vi "_io_get_StatusByte.vi"(5 "Block Setting of VISA Timeout for viReadSTB":bool, 7 "Method (viReadSTB)":u16(ring) items=["viReadSTB", "*STB?"], 8 "error in":errorcluster caption="error in (no error)", 10 "Bits filter (None - 0xFF)":u16=255 format="%.0x", 11 "VISA resource name":refnum<visa-resource-name>) -> (0 "error out":errorcluster, 1 "Error":bool, 2 "STB returned":u16 format="%.0x", 3 "VISA resource name out":refnum<visa-resource-name>, 4 "MAV":bool, 6 "OPC (ESB)":bool)   [LabVIEW 2020, in "Rohde&Schwarz RTx Oscilloscopes.lvlib" / "rsidr_core.lvlib"]
uses:
  rsidr_core.lvlib
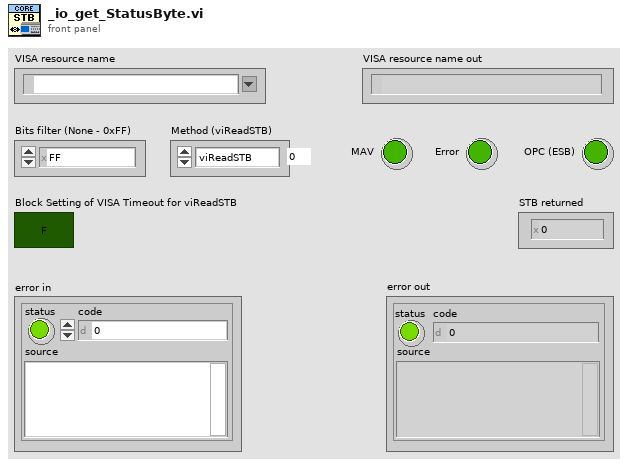
[diagram p1: front panel]
types:
  T1 = typedef "Rohde&Schwarz RTx Oscilloscopes.lvlib/rsidr_core.lvlib/type_Session_Data.ctl" = cluster{"IDN string":string, "Instrument FW":string, "Instr type":string, "Instr type for err. msg.":string, "Installed Options":string[], "Ignore Error Messages":string, "Logging params":variant, "OPC Timeout":i32, "VISA Timeout":i32, "STB Poll VISA Timeout":i32, "Additional Flags":i32, "Wait Before Read":i32, "Wait Before Write":i32, "Option String Flags":i32, "IO Segment Size":i64, "VISA Access Mode":T2, "Interface Type":T3, "OPC Wait Mode":T4, "Bin Float Number  Format":T5, "Bin Integer Number Format":T6, "Simulate":bool, "VXIcapable":bool, "Duplicate Session":bool, "Add LF to Write":bool, "Logging":bool, "Fast Sweep":bool, "Query Instrument Status":bool, "Check Range":bool, "Check Options":bool, "OPC-sync Attr Writes":bool, "OPC-sync Attr Queries":bool}
  T2 = typedef "Rohde&Schwarz RTx Oscilloscopes.lvlib/rsidr_core.lvlib/type_VisaAccessMode.ctl" = u16
  T3 = typedef "Rohde&Schwarz RTx Oscilloscopes.lvlib/rsidr_core.lvlib/type_InterfaceType.ctl" = enum16{"Unknown", "GPIB", "VXI", "GPIB_VXI", "ASRL", "PXI", "TCPIP", "USB", "SOCKET"}
  T4 = typedef "Rohde&Schwarz RTx Oscilloscopes.lvlib/rsidr_core.lvlib/type_OPC_Wait_Mode.ctl" = enum16{"STBpolling", "STBpollingSlow", "STBpollingSuperSlow", "ServiceRequest", "OPCquery"}
  T5 = typedef "Rohde&Schwarz RTx Oscilloscopes.lvlib/rsidr_core.lvlib/type_Binary_Float_Number_Format.ctl" = enum16{"Float_4_Bytes_Swapped", "Float_4_Bytes", "Double_8_Bytes_Swapped", "Double_8_Bytes"}
  T6 = typedef "Rohde&Schwarz RTx Oscilloscopes.lvlib/rsidr_core.lvlib/type_Binary_Integer_Number_Format.ctl" = enum16{"Int32_4_Bytes_Swapped", "Int32_4 Bytes", "Int16_2_Bytes_Swapped", "Int16_2_Bytes"}
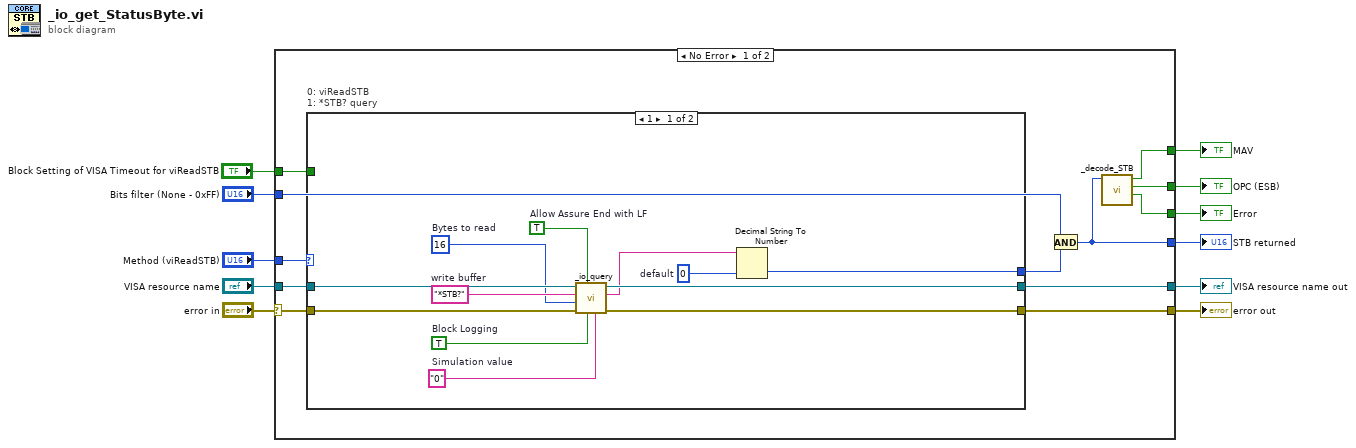
[diagram p0: block diagram]
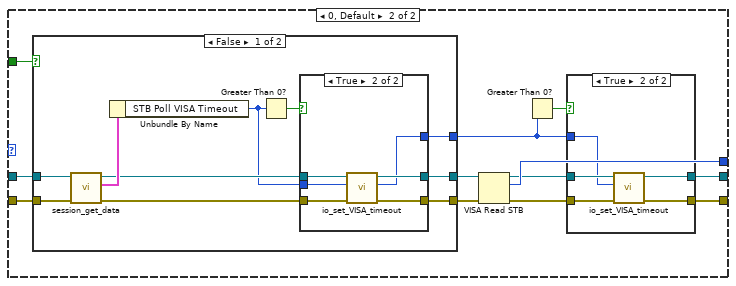
[diagram p2: hidden frame]
diagram:
  n1 = case shown="No Error" "error in" {
    selector: "error in" -> [w19 w76]
    tunnel: [w23 w76] -> w11
    tunnel: "VISA resource name" -> [w20 w75]
    tunnel: [w14 _] -> w10
    tunnel: [w21 _] -> w9
    tunnel: [w17 _] -> w8
    tunnel: [w18 _] -> w7
    tunnel: [w22 w75] -> w4
    tunnel: "Method (viReadSTB)" -> [w15 _]
    tunnel: "Bits filter (None - 0xFF)" -> [w13 _]
    tunnel: "Block Setting of VISA Timeout for viReadSTB" -> [w12 _]
    frame No Error {
      n2 = case "0: viReadSTB\n1: *STB? query" shown="1" w15 {
        tunnel: [w31 w41] -> w23
        tunnel: [w30 w36] -> w22
        tunnel: w20 -> [w32 w45]
        tunnel: w19 -> [w33 w46]
        tunnel: [w34 w47] -> w16
        tunnel: w12 -> [_ w44]
        frame 1 {
          w24 = TRUE  # Allow Assure End with LF
          w25 = "0"  # Simulation value
          w27 = TRUE  # Block Logging
          w28 = u32 16  # Bytes to read
          w35 = u16 0  # default
          w29 = "*STB?"  # write buffer
          n3 = call "_io_query.vi"("Simulation read buffer (\"Simulation\")"=w25, "Block Logging (F)"=w27, "Allow Assure End with LF"=w24, "error in"=w33, "Max bytes to read (2048)"=w28, "Write buffer"=w29, "VISA resource name"=w32) -> ("error out"=w31:errorcluster, "Read buffer"=w26:string, "VISA resource name out"=w30:refnum<visa-resource-name>)  [unwired: 1 in, 1 out]
          n4 = Decimal String To Number(string=w26, default (0L)=w35) -> (number=w34:u16)  [unwired: 1 in, 1 out]
        }
        frame 0, Default {
          n5 = case shown="False" w44 {
            tunnel: w46 -> [w64 w74]
            tunnel: w45 -> [w63 w73]
            tunnel: [w58 w74] -> w43
            tunnel: [w57 w73] -> w42
            tunnel: [w55 _] -> w37
            frame False {
              n6 = call "session_get_data.vi"("error in"=w64, "VISA resource name"=w63) -> ("error out"=w60:errorcluster, "Session User Data out"=w62:T1, "VISA resource name out"=w59:refnum<visa-resource-name>)  [unwired: 6 in, 1 out]
              n7 = Unbundle By Name(w62) -> ("STB Poll VISA Timeout"=w56:i32)
              n8 = Greater Than 0?(x=w56) -> (x > 0?=w61:bool)
              n9 = case shown="True" w61 {
                tunnel: w60 -> [w65 w72]
                tunnel: w59 -> [w66 w71]
                tunnel: [w65 w70] -> w58
                tunnel: [w66 w69] -> w57
                tunnel: w56 -> [_ w68]
                tunnel: [_ w67] -> w55
                frame False {
                }
                frame True {
                  n10 = call "io_set_VISA_timeout.vi"("error in"=w72, "VISA Timeout"=w68, "VISA resource name"=w71) -> ("error out"=w70:errorcluster, "Old VISA Timeout"=w67:u32, "VISA resource name out"=w69:refnum<visa-resource-name>)  [unwired: 6 in]
                }
              }
            }
            frame True {
            }
          }
          n11 = VISA Read STB(8:w43, 11:w42) -> (0:w40:errorcluster, 2:w47:u16, 3:w39:refnum<visa-resource-name>)
          n12 = Greater Than 0?(x=w37) -> (x > 0?=w38:bool)
          n13 = case shown="True" w38 {
            tunnel: w40 -> [w49 w54]
            tunnel: w39 -> [w48 w53]
            tunnel: [w49 w52] -> w41
            tunnel: [w48 w51] -> w36
            tunnel: w37 -> [_ w50]
            frame False {
            }
            frame True {
              n14 = call "io_set_VISA_timeout.vi"("error in"=w54, "VISA Timeout"=w50, "VISA resource name"=w53) -> ("error out"=w52:errorcluster, "VISA resource name out"=w51:refnum<visa-resource-name>)  [unwired: 6 in, 1 out]
            }
          }
        }
      }
      n15 = And(x=w13, y=w16) -> (x .and. y?=w14:u16)
      n16 = call "_decode_STB.vi"("STB in"=w14) -> ("Error"=w17:bool, "OPC (ESB)"=w18:bool, "MAV"=w21:bool)  [unwired: 7 in, 1 out]
    }
    frame Error {
    }
  }
  "VISA resource name out" <- w4
  "error out" <- w11
  "STB returned" <- w10
  "MAV" <- w9
  "Error" <- w8
  "OPC (ESB)" <- w7
